vi "SCD - Externally Triggered Image Acquisition - v2.vi"(0 "FPS":dbl=10.0 format="%0.2p", 1 "LCVR Voltages":dbl[][](array[numeric]), 5 "Modulation Cycles":i32=1 min=1 max=30 step=1, 9 "Headers In":T4[](array[typedef])=[{"Wavelength (nm)"=530.15, "Exposure (s)"=0.05, "Tuning Delay (ms)"=1000.0, "Beam Type (-1/1)"=1.0, "Tuning Voltages"=[1.111, 2.222, 3.333, 4.444], "Observer"="observer", "Light Shapping Diffuser"=enum."In Beam", "Comment"="", "Data Type"=9, "Mod Cycles"=0, "SCD Calibration Optics"=enum."1 - Polarizer @0, I+Q", "SCD Emission Line Filter"=enum."1-557.6nm", "Cookbook"="", "COMP-S Calibration Wheel"=enum."Dark", "COMP-S Andover Filter Wheel"=enum."530.3nm/HWB 0.34nm (Fe XIV)", "FOV Rotation (deg)"=66.0, "Objective Lens Position (mm)"=0.0, "Occulter size"=0.0, "Time End"=timestamp(3382374145.421875 s since 1904-01-01), "Acc Exposure (s)"=0.0, "Time Stamp Array"=[], "Camera Serial Number"=[], "Camera Temp"=[], "Camera PI (mm)"=[0.0, 0.0, 0.0], "Time Start"=timestamp(3382374145.421875 s since 1904-01-01), "Peripherals"={"ILX controler"=FALSE, "Zone temperatures"=FALSE, "Andor"=FALSE, "Andor 2"=FALSE, "PI Stage"=FALSE, "AISAS mechanisms"=FALSE, "AISAS Mech.lvclass"=refnum, "Zone temp ref"=variant, "FW"=FALSE}}] {"Camera PI (mm)" format="%_3g"; "Acc Exposure (s)" format="%^.3g"; "Occulter size" format="%.2f"; "Objective Lens Position (mm)" min=70.0 max=152.0 format="%.2f"; "FOV Rotation (deg)" format="%.1f"; "Data Type" items=["LIVE", "DARK", "FLAT", "CALI", "OBSE", "ABSO", "AURE", "TARG", "OBJE", "HOLE", "OREX", "THRO", "CHIP"]; "Exposure (s)" format="%^.3g"; "Wavelength (nm)" format="%_6g"}, 11 "error in":errorcluster, 12 "Neo Info":T2={"Handle"=104, "Pixel Encoding"="Mono16", "AOI Width"=2560, "AOI Height"=2160, "AOI Stride"=5136, "Image Bytes"=11098896, "Image Pixels"=5529600, "Row Readout Time"=9.371428571428572e-06, "Frame Readout Time"=0.010121142857142858, "Interframe Time"=8.434285714285715e-05, "Semaphore"=refnum, "SerialNumber"="SCC-02209", "Camera Model"="DC-152Q-C00-FI", "Controller ID"="3", "Firmware Version"="13.8.26.122", "Shutter"="Global", "Binning"=0, "Time at Synch"=timestamp(3029526000.379448 s since 1904-01-01), "Idx"=0} {"Time at Synch" format="%<%H:%M:%S>T"; "Interframe Time" format="%#_3g"; "Frame Readout Time" format="%_3g"; "Row Readout Time" format="%_3g"}, 14 "Timestamp at Synch":timestamp) -> (3 "FITS Path Out":path, 4 "Andor Handle Out":i32, 6 "Most Recent Image Accumulation (Modulation State A)":u32[][](graph), 10 "Headers Out":T4[](array[typedef]) {"Camera PI (mm)" format="%_3g"; "Acc Exposure (s)" format="%^.3g"; "Occulter size" format="%.2f"; "Objective Lens Position (mm)" min=70.0 max=152.0 format="%.2f"; "FOV Rotation (deg)" format="%.1f"; "Data Type" items=["LIVE", "DARK", "FLAT", "CALI", "OBSE", "ABSO", "AURE", "TARG", "OBJE", "HOLE", "OREX", "THRO", "CHIP"]; "Exposure (s)" format="%^.3g"; "Wavelength (nm)" format="%_6g"}, 15 "error out":errorcluster={"status"=FALSE, "code"=5000, "source"="AT Finalise Library A.vi\n\nSUCCESS"})   [LabVIEW 2014]
doc: "The LL Sequence VI acquires a sequence of images and displays them in an array of image controls using the low-level acquisition VIs. A sequence is appropriate for applications that process multiple images. You can configure a sequence to acquire every frame or to skip a variable number of frames between each image.\n\nTop Level Code Overview\n1) Initialize Camera (Global Shutter, High Well, Low Noise, exposure time, etc.)\n2) Create a buffer set equal in size to the # of trigger pulses (e.g. 100) which is the same as the # of expected images \n3) Start the camera acquisition THEN start the DAQmx task (use merge error cluster to gurantee this)"
uses:
  <vilib>/DAQmx/configure/timing.llb/DAQmx Timing (Use Waveform).vi
  <vilib>/DAQmx/create/channels.llb/DAQmx Create Channel (AO-Voltage-Basic).vi
  <vilib>/DAQmx/write.llb/DAQmx Write (Analog 1D Wfm NChan NSamp).vi
  <vilib>/Waveform/WDTOps.llb/WDT Waveform Duration DBL.vi
  Controls/SCD - Calibration Optics Filter Wheel.ctl
  AISAS/Controls/Diffuser.ctl
  Controls/SCD - FITS Cluster.ctl
  Camera/Andor Neo Info.ctl
  Controls/SCD - EDT - Emission Line Filter Wheel.ctl
  Controls/CoMP-S Controls/Polarization Optics Filter Wheel.ctl
  Controls/CoMP-S Controls/Emission Line Filter Wheel.ctl
  AISAS/Controls/focus.ctl
  AISAS/Mech/AISAS Mech.lvclass
  Controls/peripherals.ctl
panel:
  in  "Tab Control":T1(tab)
  in  "Save to FITS":bool=TRUE
  out "# images to acquire":i32
  out "SCD Waveforms":waveform(dbl)[](graph)
  out "Image Acquisition Started":bool
  out "PixelData [U16]":u16[](array[numeric])
  out "ByteData [U8]":u8[](array[numeric])
  out "Andor Handle In":i32=104
  in  "image pointers":u64[](array[numeric])
  in  "imageNo":i32
  in  "count":i32
  out "Acquisition Estimate (s)":dbl=0.6002500000000001 format="%0.2f"
  out "# Wavelengths":i32=1
  out "Exposure Get (s)":dbl=0.09
  out "Image Acq (s)":dbl(slide)=4151.832132564842
  out "# elements in queue":i32
  out "COMP Waveforms":waveform(dbl)[](graph)
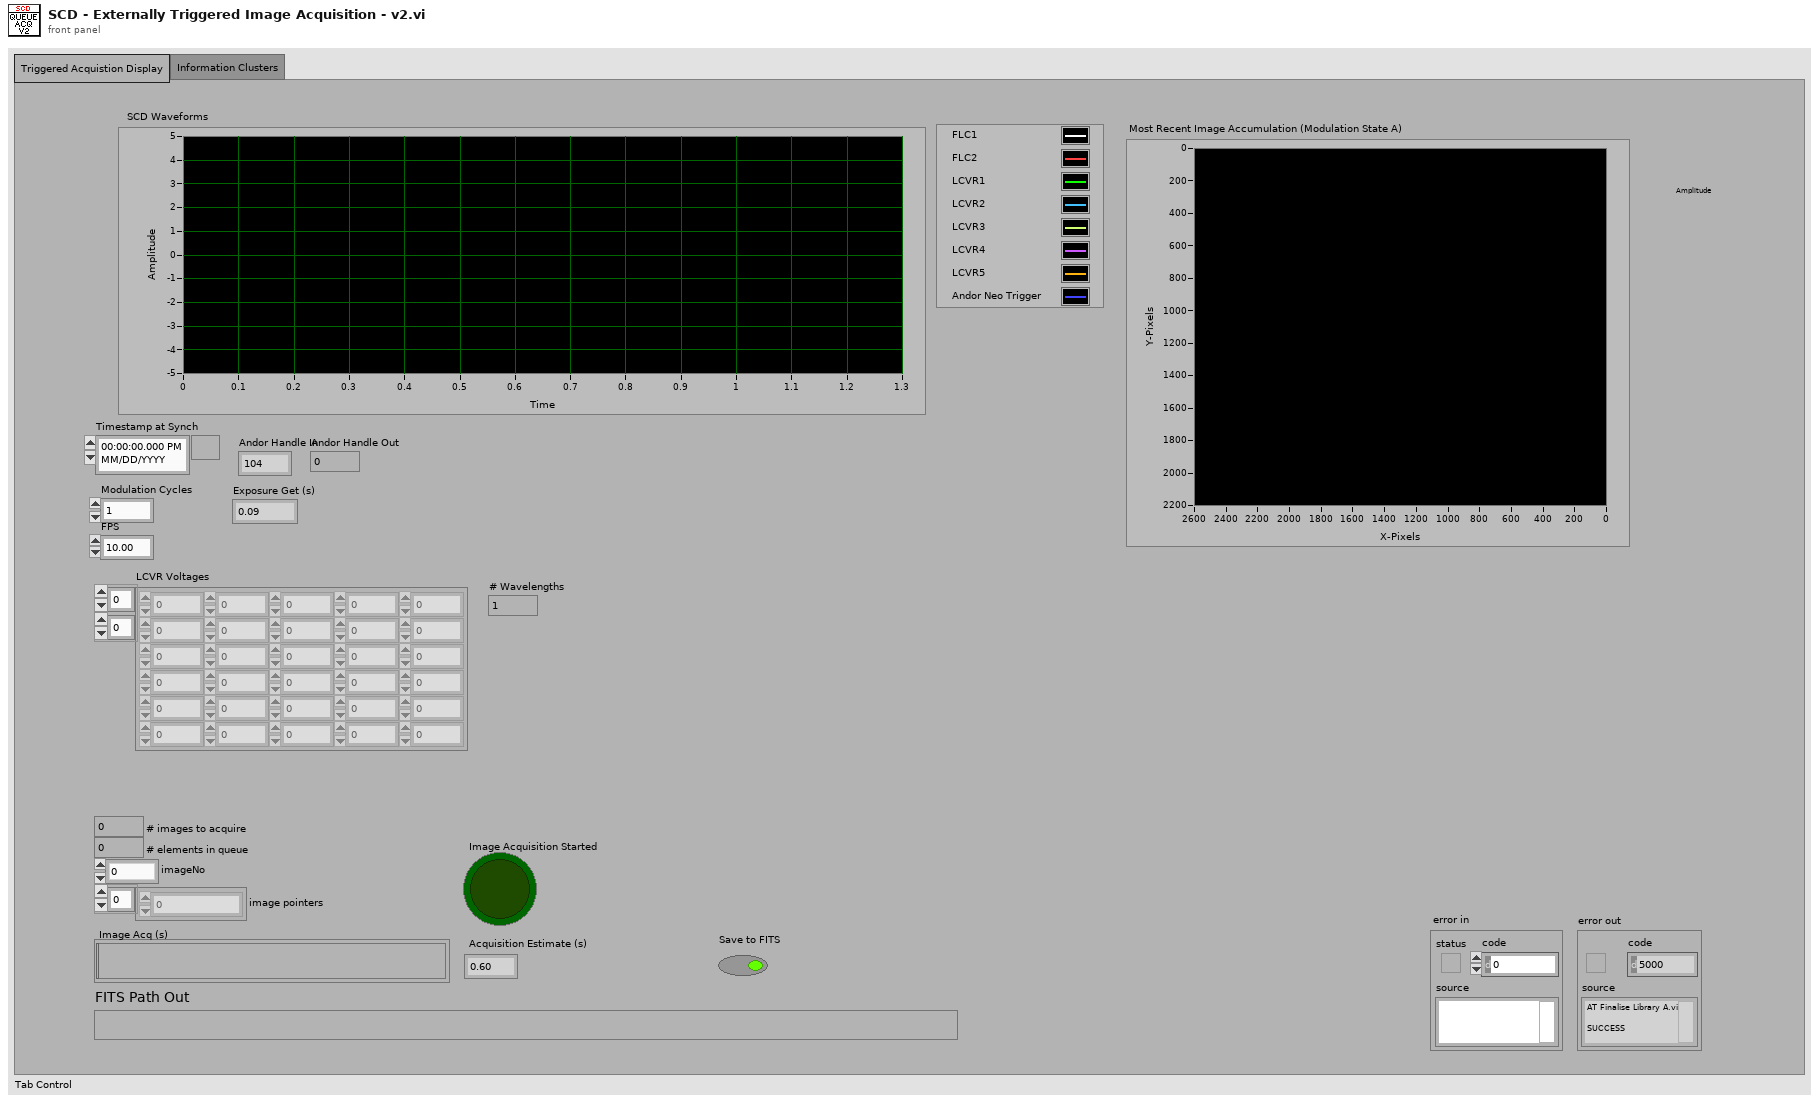
[diagram p1: front panel]
types:
  T1 = enum32{"Triggered Acquistion Display", "Information Clusters"}
  T2 = typedef "Andor Neo Info.ctl" = cluster{"Handle":i32, "Pixel Encoding":string, "AOI Width":i64, "AOI Height":i64, "AOI Stride":i64, "Image Bytes":i64, "Image Pixels":i64, "Row Readout Time":dbl, "Frame Readout Time":dbl, "Interframe Time":dbl, "Semaphore":T3, "SerialNumber":string, "Camera Model":string, "Controller ID":string, "Firmware Version":string, "Shutter":string, "Binning":u8, "Time at Synch":timestamp, "Idx":i32}
  T3 = typedef "Semaphore RefNum" = refnum<k1>
  T4 = typedef "SCD - FITS Cluster.ctl" = cluster{"Wavelength (nm)":dbl, "Exposure (s)":dbl, "Tuning Delay (ms)":dbl, "Beam Type (-1/1)":dbl, "Tuning Voltages":dbl[], "Observer":string, "Light Shapping Diffuser":T5, "Comment":string, "Data Type":u16, "Mod Cycles":u16, "SCD Calibration Optics":T6, "SCD Emission Line Filter":T7, "Cookbook":string, "COMP-S Calibration Wheel":T8, "COMP-S Andover Filter Wheel":T9, "FOV Rotation (deg)":dbl, "Objective Lens Position (mm)":T10, "Occulter size":dbl, "Time End":timestamp, "Acc Exposure (s)":dbl, "Time Stamp Array":timestamp[], "Camera Serial Number":string[], "Camera Temp":dbl[], "Camera PI (mm)":dbl[], "Time Start":timestamp, "Peripherals":T11}
  T5 = typedef "Diffuser.ctl" = enum16{"Out of Beam", "In Beam"}
  T6 = typedef "SCD - Calibration Optics Filter Wheel.ctl" = enum16{"1 - Polarizer @0, I+Q", "2 - Polarizer @90, I-Q", "3 - Polarizer @45, I+U", "4 - Polarizer @135, I-U", "5 - Polarizer @0, Retarder @45, I+V", "6 - Polarizer @0, Retarder @135, I-V", "7 - Dark", "8 - Clear", "9 - N/A"}
  T7 = typedef "SCD - EDT - Emission Line Filter Wheel.ctl" = enum16{"1-557.6nm", "2-587.6nm", "3-589.6nm", "4-630.2nm", "5-656.4nm", "6-849.8nm", "7-854.2nm", "8-866.2nm", "9-1083.0nm"}
  T8 = typedef "Polarization Optics Filter Wheel.ctl" = enum16{"Dark", "Clear", "Exchange Lens", "Polarizer @0, I+Q", "Polarizer @90, I-Q", "Polarizer @45, I+U", "Polarizer @135, I-U", "Polarizer @0, Retarder @45, I+V", "Polarizer @0, Retarder @135, I-V"}
  T9 = typedef "Emission Line Filter Wheel.ctl" = enum16{"530.3nm/HWB 0.34nm (Fe XIV)", "587.6nm/HBW 0.44nm (He I D3)", "637.5nm/HBW 0.53nm (Fe X)", "656.3nm/HBW 0.57nm (H-Alpha)", "789.2nm/HBW 0.85nm (Fe XI)", "854.2nm/HBW 1.01nm (Ca I)", "1074.7nm/HBW 2.34nm (Fe XIII)", "1079.8nm/HBW 1.64nm (Fe XIII)", "1083.0nm/HBW 1.66nm (He I)"}
  T10 = typedef "focus.ctl" = dbl
  T11 = typedef "peripherals.ctl" = cluster{"ILX controler":bool, "Zone temperatures":bool, "Andor":bool, "Andor 2":bool, "PI Stage":bool, "AISAS mechanisms":bool, "AISAS Mech.lvclass":refnum<class "AISAS Mech.lvclass">, "Zone temp ref":variant, "FW":bool}
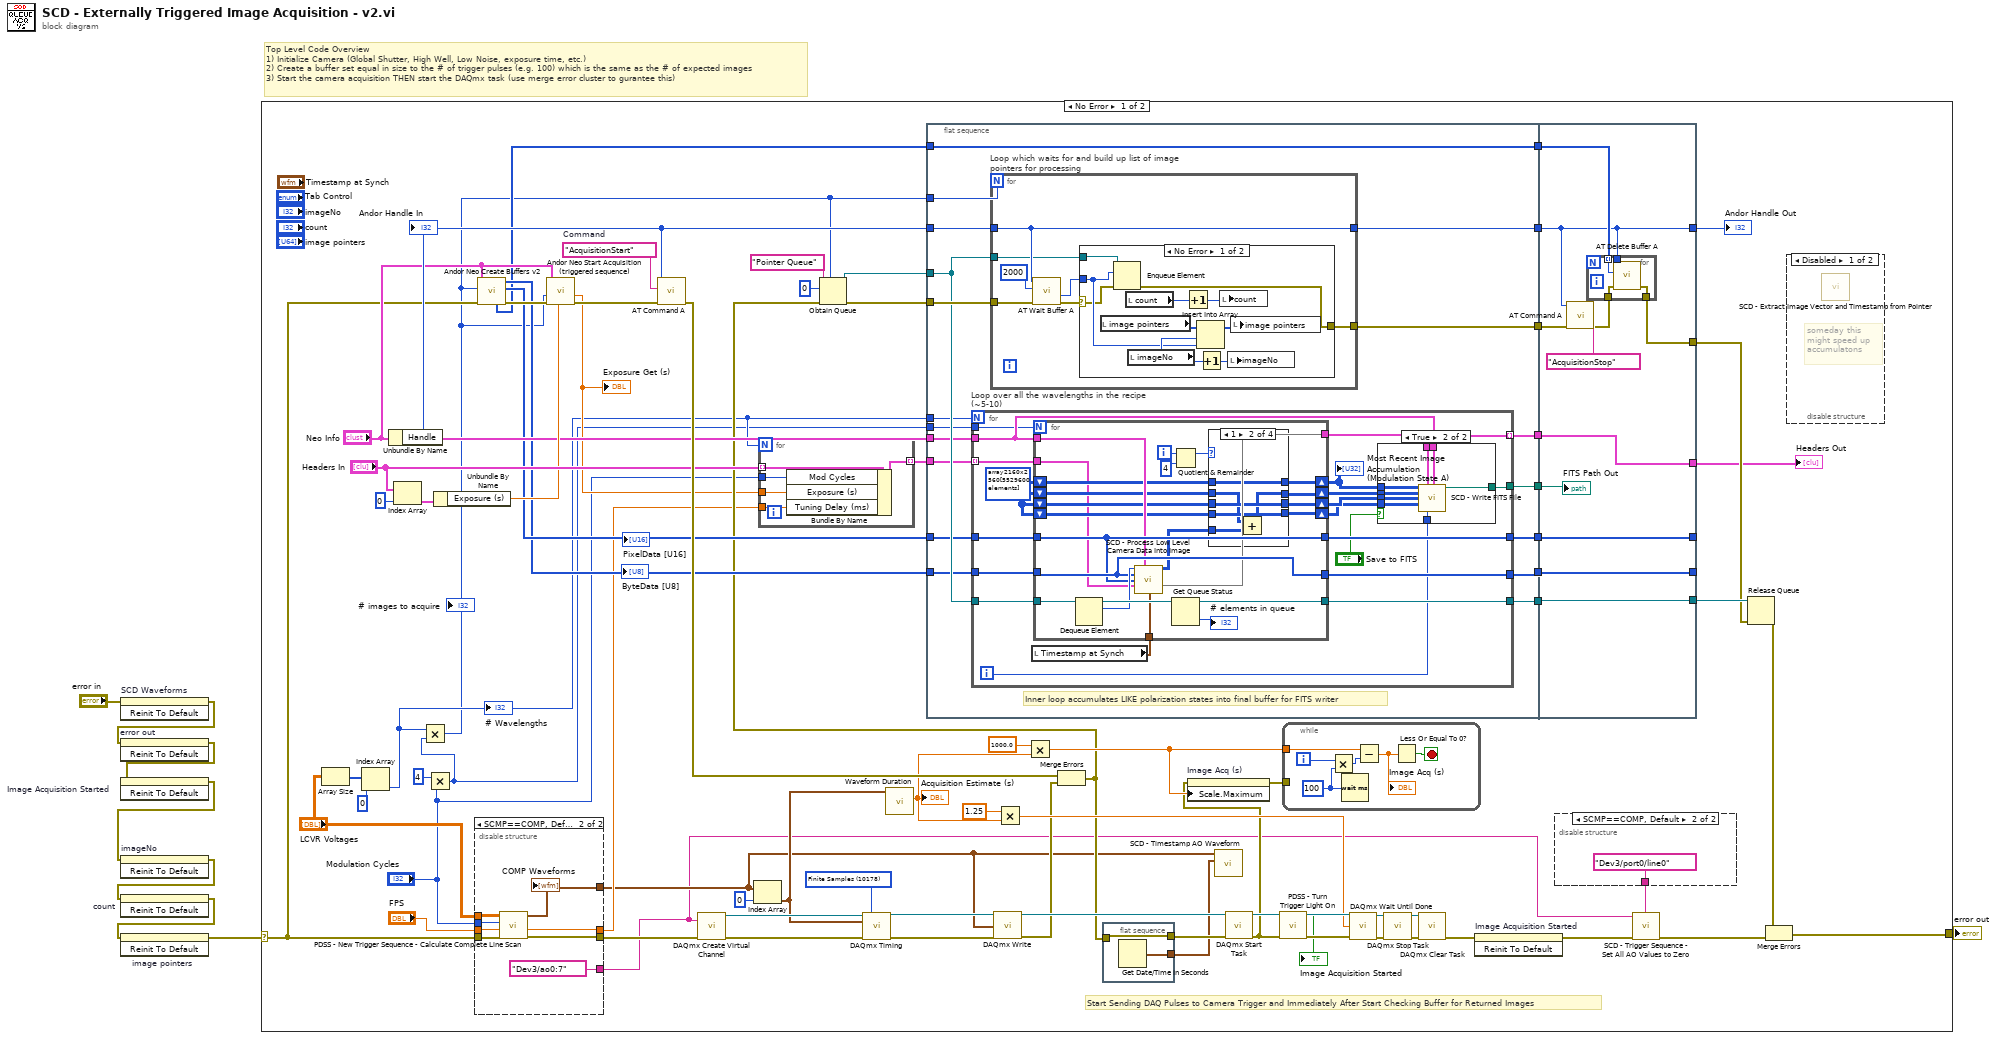
[diagram p0: block diagram]
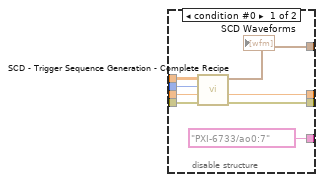
[diagram p2: hidden frame]
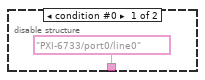
[diagram p3: hidden frame]
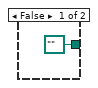
[diagram p5: hidden frame]
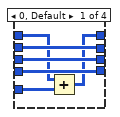
[diagram p6: hidden frame]
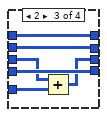
[diagram p7: hidden frame]
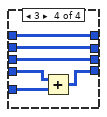
[diagram p8: hidden frame]
diagram:
  # "Top Level Code Overview\n1) Initialize Camera (Global Shutter, High Well, Low Noise, exposure time, etc.)\n2) Create a buffer set equal in size to the # of trigger pulses (e.g. 100) which is the same as the # of expected images \n3) Start the camera acquisition THEN start the DAQmx task (use merge error cluster to gurantee this)"
  n1 = invoke on="SCD Waveforms" class="WFGraph (strict)" method="Reinit To Default"(error in="error in") -> (error out=w6:errorcluster)  [unwired: 2 in, 2 out]
  n2 = invoke on="error out" class="Clust (strict)" method="Reinit To Default"(error in=w6) -> (error out=w5:errorcluster)  [unwired: 2 in, 2 out]
  n3 = invoke on="Image Acquisition Started" class="Bool (strict)" method="Reinit To Default"(error in=w5) -> (error out=w1:errorcluster)  [unwired: 2 in, 2 out]
  n4 = invoke on="imageNo" class="DigNum (strict)" method="Reinit To Default"(error in=w1) -> (error out=w4:errorcluster)  [unwired: 2 in, 2 out]
  n5 = invoke on="count" class="DigNum (strict)" method="Reinit To Default"(error in=w4) -> (error out=w3:errorcluster)  [unwired: 2 in, 2 out]
  n6 = invoke on="image pointers" class="Arr (strict)" method="Reinit To Default"(error in=w3) -> (error out=w2:errorcluster)  [unwired: 2 in, 2 out]
  n7 = case shown="No Error" w2 {
    selector: w2 -> [w27 w243]
    tunnel: [w56 w243] -> w8
    frame No Error {
      w61 = "AcquisitionStart"  # Command
      w85 = 10178 items=["Finite Samples"=10178, "Continuous Samples"=10123] ("sample mode")
      # "Start Sending DAQ Pulses to Camera Trigger and Immediately After Start Checking Buffer for Returned Images"
      n8 = Array Size(array="LCVR Voltages") -> (size(s)=w67:i32[])
      n9 = Index Array(array=w67, index=0) -> (element=w15:i32)
      "# Wavelengths" <- w15
      n10 = Unbundle By Name("Neo Info") -> ("Handle"=w55:i32)
      "Andor Handle In" <- w55
      n11 = Index Array(array="Headers In", index=0) -> (element=w47:T4)
      n12 = Multiply(x=4 ("value"), y="Modulation Cycles") -> (x*y=w14:i32)
      n13 = Multiply(x=w15, y=w14) -> (x*y=w13:i32)
      "# images to acquire" <- w13
      n14 = Unbundle By Name(w47) -> ("Exposure (s)"=w46:dbl)
      n15 = disable-structure shown="SCMP==COMP, Default" {
        disable-tunnel: [w93 w97] -> w75
        disable-tunnel: "LCVR Voltages" -> [w92 w101]
        disable-tunnel: [w87 w94] -> w10
        disable-tunnel: "FPS" -> [w91 w99]
        disable-tunnel: w27 -> [w90 w98]
        disable-tunnel: [w89 w96] -> w17
        disable-tunnel: "Modulation Cycles" -> [w88 w100]
        disable-tunnel: [tag "PXI-6733/ao0:7" ("physical channels") tag "Dev3/ao0:7" ("physical channels")] -> w9
        frame condition #0 {
          n16 = call "SCD - Trigger Sequence Generation - Complete Recipe.vi"("error in"=w90, "FPS"=w91, "Modulation Cycles\nAt Each Wavelength"=w88, "LCVR Voltages"=w92) -> ("error out"=w93:errorcluster, "LCVR Relaxtion Time"=w89:dbl, "SCD Waveforms (Graph)"=w87:waveform(dbl)[])  [unwired: 5 in]
          "SCD Waveforms" <- w87
        }
        frame condition #1 (active) {
          n17 = call "PDSS - New Trigger Sequence - Calculate Complete Line Scan.vi"("error in"=w98, "FPS"=w99, "Modulation Cycles\nAt Each Wavelength"=w100, "LCVR Voltages"=w101) -> ("error out"=w97:errorcluster, "LCVR Relaxtion Time"=w96:dbl, "AO Graph"=w94:waveform(dbl)[])  [unwired: 5 in]
          "COMP Waveforms" <- w94
        }
      }
      n18 = call "Andor Neo Create Buffers v2.vi"("error in"=w27, "Number of Buffers"=w13, "Camera Info"="Neo Info") -> ("error out"=w54:errorcluster, "PixelData"=w40:i64[], "ByteData"=w38:u8[], "Array of Buffers"=w19:u64[])  [unwired: 5 in]
      "ByteData [U8]" <- w38
      "PixelData [U16]" <- w40
      n19 = call "Andor Neo Start Acquisition (triggered sequence).vi"("Exposure Set (s)"=w46, "error in"=w54, "Frames"=w13, "Camera Info"="Neo Info") -> ("error out"=w44:errorcluster, "Exposure Get (s)"=w16:dbl)  [unwired: 6 in]
      "Exposure Get (s)" <- w16
      n20 = call <userlib>:"AT Command A.vi"("error in (no error)"=w44, "Feature"=w61, "Handle"=w55) -> ("error out"=w53:errorcluster)  [unwired: 7 in, 1 out]
      n21 = call-poly <vilib>:"DAQmx Create Virtual Channel.vi"("physical channels"=w9, "error in"=w75) -> ("task out"=w82:refnum<k21>, "error out"=w83:errorcluster)  [unwired: 12 in]
      n22 = Index Array(array=w10, index=0) -> (element=w72:waveform(dbl))
      n23 = for {
        N: w15 -> [_]
        tunnel: [w114] -> w42 mode=indexing
        tunnel: w16 -> [w113]
        tunnel: "Headers In" -> [w112] mode=indexing
        tunnel: w17 -> [w111]
        tunnel: "Modulation Cycles" -> [w110]
        n24 = Bundle By Name(cluster=w112, "Mod Cycles"=w110, "Exposure (s)"=w113, "Tuning Delay (ms)"=w111) -> (w114:T4)
      }
      n25 = call-poly <vilib>:"DAQmx Timing.vi"("task/channels in"=w82, "sample mode"=w85, "waveform"=w72, "error in"=w83) -> ("task out"=w73:refnum<k21>, "error out"=w74:errorcluster)  [unwired: 10 in]
      n26 = call-poly <vilib>:"Waveform Duration.vi"("waveform in"=w72) -> ("duration"=w30:dbl)  [unwired: 8 in, 2 out]
      "Acquisition Estimate (s)" <- w30
      n27 = flat-sequence {
        tunnel: w35 -> [w134]
        tunnel: w13 -> [w122]
        tunnel: w55 -> [w133]
        tunnel: [w132] -> w60
        tunnel: [w131] -> w59
        tunnel: "Neo Info" -> [w123]
        tunnel: w42 -> [w125]
        tunnel: [w124] -> w41
        tunnel: w40 -> [w126]
        tunnel: [w121] -> w39
        tunnel: w38 -> [w129]
        tunnel: [w127] -> w37
        tunnel: w34 -> [w130]
        tunnel: [w128] -> w32
        tunnel: w15 -> [w120]
        tunnel: [w119] -> w26
        tunnel: w19 -> [w118]
        tunnel: [w118] -> w18
        tunnel: w14 -> [w117]
        tunnel: w60 -> [w231]
        tunnel: w59 -> [w237]
        tunnel: [w231] -> w52
        tunnel: [w229] -> w23
        tunnel: [w236] -> w22
        tunnel: w41 -> [w236]
        tunnel: [w235] -> _
        tunnel: w39 -> [w235]
        tunnel: [w234] -> _
        tunnel: w37 -> [w234]
        tunnel: w32 -> [w233]
        tunnel: [w233] -> w31
        tunnel: w26 -> [w228]
        tunnel: w18 -> [w232]
        frame #0 {
          # "Inner loop accumulates LIKE polarization states into final buffer for FITS writer"
          n28 = for "Loop over all the wavelengths in the recipe (~5-10)" {
            N: w120 -> [_]
            tunnel: w130 -> [w153]
            tunnel: w129 -> [w152]
            tunnel: [w151] -> w128
            tunnel: [w150] -> w127
            tunnel: w126 -> [w149]
            tunnel: w125 -> [w148] mode=indexing
            tunnel: [w140] -> w124 mode=indexing
            tunnel: w123 -> [w138]
            tunnel: [w143] -> w121
            tunnel: [w142] -> w119
            tunnel: w117 -> [w137]
            i -> [w136]
            w147 = i32[][] array2160x2560[5529600 elements] ("2560x2160 Initialized Array")
            n29 = local read "Timestamp at Synch"() -> (w141:timestamp)
            n30 = for {
              N: w137 -> [_]
              tunnel: w153 -> [w185]
              tunnel: w152 -> [w182]
              tunnel: [w167] -> w151
              tunnel: [w182] -> w150
              tunnel: w149 -> [w181]
              tunnel: [w181] -> w143
              tunnel: w148 -> [w165]
              tunnel: [w164] -> w140
              tunnel: w138 -> [w180]
              shift-right: [w172] -> w139
              shift-left: w147 -> [w173]
              shift-right: [w171] -> w146
              shift-left: w147 -> [w174]
              shift-right: [w170] -> w145
              shift-left: w147 -> [w175]
              shift-right: [w169] -> w144
              shift-left: w147 -> [w176]
              tunnel: w141 -> [w163]
              i -> [w178]
              n31 = Dequeue Element(queue=w185) -> (queue out=w184:refnum<queue>, element=w183:u64)  [unwired: 2 in, 2 out]
              n32 = call "SCD - Process Low Level Camera Data Into Image.vi"("Pointer In"=w183, "Neo Info"=w180, 2:w163, "ByteData (U8)"=w182, "PixelData (U16)"=w181, 9:w165) -> ("Image (I32)"=w168:u32[][], 10:w164)  [unwired: 6 in, 2 out]
              n33 = Quotient & Remainder(x=w178, y=4) -> (x-y*floor(x/y)=w177:i32)  [unwired: 1 out]
              n34 = Get Queue Status(queue=w184) -> (queue out=w167:refnum<queue>, # elements in queue=→"# elements in queue":i32)  [unwired: 2 in, 6 out]
              n35 = case shown="1" w177 {
                tunnel: w176 -> [w189 w196 w202 w205]
                tunnel: w175 -> [w190 w197 w199 w208]
                tunnel: w174 -> [w191 w193 w203 w209]
                tunnel: w173 -> [w187 w194 w200 w206]
                tunnel: [w186 w194 w200 w206] -> w172
                tunnel: [w191 w192 w203 w209] -> w171
                tunnel: [w190 w197 w198 w208] -> w170
                tunnel: [w189 w196 w202 w204] -> w169
                tunnel: w168 -> [w188 w195 w201 w207]
                frame 0, Default {
                  n36 = Add(x=w187, y=w188) -> (x+y=w186:u32[][])
                }
                frame 1 {
                  n37 = Add(x=w193, y=w195) -> (x+y=w192:u32[][])
                }
                frame 2 {
                  n38 = Add(x=w199, y=w201) -> (x+y=w198:u32[][])
                }
                frame 3 {
                  n39 = Add(x=w205, y=w207) -> (x+y=w204:u32[][])
                }
              }
            }
            "Most Recent Image Accumulation (Modulation State A)" <- w139
            n40 = case shown="True" "Save to FITS" {
              tunnel: w146 -> [_ w162]
              tunnel: w145 -> [_ w161]
              tunnel: w144 -> [_ w160]
              tunnel: [path "" ("FITS Path Out") w159] -> w142
              tunnel: w140 -> [_ w158]
              tunnel: w139 -> [_ w157]
              tunnel: w138 -> [_ w156]
              tunnel: w136 -> [_ w155]
              frame False {
              }
              frame True {
                n41 = call "SCD - Write FITS File.vi"("A"=w157, "FITS Header"=w158, "Neo Info"=w156, "B"=w162, "C"=w161, "D"=w160, "Image #"=w155) -> ("FITS Path Out"=w159:path)  [unwired: 6 in, 2 out]
              }
            }
          }
          n42 = for "Loop which waits for and build up list of image pointers for processing" {
            N: w122 -> [_]
            tunnel: w133 -> [w213]
            tunnel: w134 -> [w215]
            tunnel: [w213] -> w132
            tunnel: [w211] -> w131
            tunnel: w130 -> [w210]
            n43 = call <userlib>:"AT Wait Buffer A.vi"("error in (no error)"=w215, "Timeout"=u32 2000, "Handle"=w213) -> ("error out"=w212:errorcluster, "Output buffer"=w214:u64)  [unwired: 5 in, 2 out]
            n44 = case shown="No Error" w212 {
              selector: w212 -> [w218 w227]
              tunnel: w214 -> [w220 _]
              tunnel: [w217 w227] -> w211
              tunnel: w210 -> [w219 _]
              frame No Error {
                n45 = local read "image pointers"() -> (w224:u64[])
                n46 = Enqueue Element(queue=w219, element=w220, error in (no error)=w218) -> (error out=w217:errorcluster)  [unwired: 1 in, 2 out]
                n47 = local read "count"() -> (w226:i32)
                n48 = local read "imageNo"() -> (w221:i32)
                n49 = Increment(x=w226) -> (x+1=w225:i32)
                n50 = Insert Into Array(array=w224, index=w221, new element=w220) -> (w223:u64[])
                n51 = Increment(x=w221) -> (x+1=w222:i32)
                n52 = local write "count"(w225) -> ()
                n53 = local write "imageNo"(w222) -> ()
                n54 = local write "image pointers"(w223) -> ()
              }
              frame Error {
              }
            }
          }
        }
        frame #1 {
          n55 = call <userlib>:"AT Command A.vi"("error in (no error)"=w237, "Feature"="AcquisitionStop" ("Command"), "Handle"=w231) -> ("error out"=w230:errorcluster)  [unwired: 7 in, 1 out]
          n56 = for {
            tunnel: w232 -> [w242] mode=indexing
            tunnel: w231 -> [w241]
            tunnel: w230 -> [w240]
            tunnel: [w239] -> w229
            n57 = call <userlib>:"AT Delete Buffer A.vi"("error in (no error)"=w240, "Buffer"=w242, "Handle"=w241) -> ("error out"=w239:errorcluster)  [unwired: 7 in, 1 out]
          }
          "FITS Path Out" <- w228
        }
      }
      n58 = call-poly <vilib>:"DAQmx Write.vi"("task/channels in"=w73, "data"=w10, "error in"=w74) -> ("task out"=w84:refnum<k21>, "error out"=w58:errorcluster)  [unwired: 10 in, 1 out]
      n59 = Multiply(x=1.25, y=w30) -> (x*y=w63:dbl)
      n60 = Multiply(x=1000.0, y=w30) -> (x*y=w28:dbl)
      n61 = Merge Errors(w53, w58) -> (w24:errorcluster)
      n62 = Obtain Queue(max queue size (-1, unlimited)=w13, name (unnamed)="Pointer Queue", element data type=u64 0 ("Output buffer"), error in (no error)=w24) -> (queue out=w34:refnum<queue>, error out=w35:errorcluster)  [unwired: 1 in, 1 out]
      n63 = flat-sequence {
        tunnel: [w116] -> w51
        tunnel: w24 -> [w116]
        tunnel: [w115] -> w50
        frame #0 {
          n64 = Get Date/Time In Seconds() -> (seconds since 1Jan1904=w115:timestamp)
        }
      }
      n65 = call "SCD - Timestamp AO Waveform.vi"("DAQ To"=w50, "SCD AO Waveforms"=w10) -> ()  [unwired: 8 in, 2 out]
      n66 = call <vilib>:"DAQmx Start Task.vi"("task/channels in"=w84, "error in"=w51) -> ("task out"=w81:refnum<k21>, "error out"=w21:errorcluster)  [unwired: 12 in]
      n67 = property on="Image Acq (s)" class="Slide (strict)"(error in=w21, "Scale.Maximum"=w28) -> (error out=w20:errorcluster)  [unwired: 1 in, 1 out]
      n68 = call "PDSS - Turn Trigger Light On.vi"("error in (no error)"=w21) -> ("error out"=w70:errorcluster, "Trigger Started"=→"Image Acquisition Started":bool)  [unwired: 9 in]
      n69 = while {
        tunnel: w28 -> [w108]
        tunnel: w20 -> [_]
        i -> [w106]
        stop <- w107 stop-if-true
        w105 = u32 100 ("milliseconds to wait")
        n70 = Multiply(x=w106, y=w105) -> (x*y=w109:u32)
        n71 = Wait (ms)(milliseconds to wait=w105) -> ()  [unwired: 1 out]
        n72 = Subtract(x=w108, y=w109) -> (x-y=w104:dbl)
        "Image Acq (s)" <- w104
        n73 = Less Or Equal To 0?(x=w104) -> (x <= 0?=w107:bool)
      }
      n74 = call <vilib>:"DAQmx Wait Until Done.vi"("task/channels in"=w81, "timeout (sec)"=w63, "error in"=w70) -> ("task out"=w80:refnum<k21>, "error out"=w79:errorcluster)  [unwired: 11 in]
      n75 = call <vilib>:"DAQmx Stop Task.vi"("task/channels in"=w80, "error in"=w79) -> ("task out"=w78:refnum<k21>, "error out"=w77:errorcluster)  [unwired: 12 in]
      n76 = call <vilib>:"DAQmx Clear Task.vi"("task in"=w78, "error in"=w77) -> ("error out"=w65:errorcluster)  [unwired: 13 in]
      n77 = invoke on="Image Acquisition Started" class="Bool (strict)" method="Reinit To Default"(error in=w65) -> (error out=w64:errorcluster)  [unwired: 2 in, 2 out]
      n78 = disable-structure shown="SCMP==COMP, Default" {
        disable-tunnel: [tag "PXI-6733/port0/line0" ("lines") tag "Dev3/port0/line0" ("lines")] -> w62
        frame condition #0 {
        }
        frame condition #1 (active) {
        }
      }
      n79 = call "SCD - Trigger Sequence - Set All AO Values to Zero.vi"("error in"=w64, "lines"=w62, "physical channels"=w9) -> ("error out"=w57:errorcluster)  [unwired: 8 in]
      n80 = Release Queue(queue=w31, error in (no error)=w23) -> (error out=w25:errorcluster)  [unwired: 1 in, 2 out]
      n81 = Merge Errors(w25, w57) -> (w56:errorcluster)
      n82 = disable-structure shown="Disabled" {
        frame Disabled {
          # "someday this\nmight speed up\naccumulatons"
          n83 = call "SCD - Extract Image Vector and Timestamp from Pointer.vi"() -> ()  [unwired: 13 in, 3 out]
        }
        frame Enabled {
        }
      }
      "Andor Handle Out" <- w52
      "Headers Out" <- w22
    }
    frame Error {
    }
  }
  "error out" <- w8
